vi "XDSBMPread.vi"() -> ()   [LabVIEW 2013]
panel:
  out "new picture":picture caption="new bmp"
  in  "stop":bool
  in  "base path":path=path "C:/Users/Administrator/Desktop/新建文件夹 (2)"
  in  "file name":string="a"
  # "1.This vi can read the picture of the osc screen by LAN"
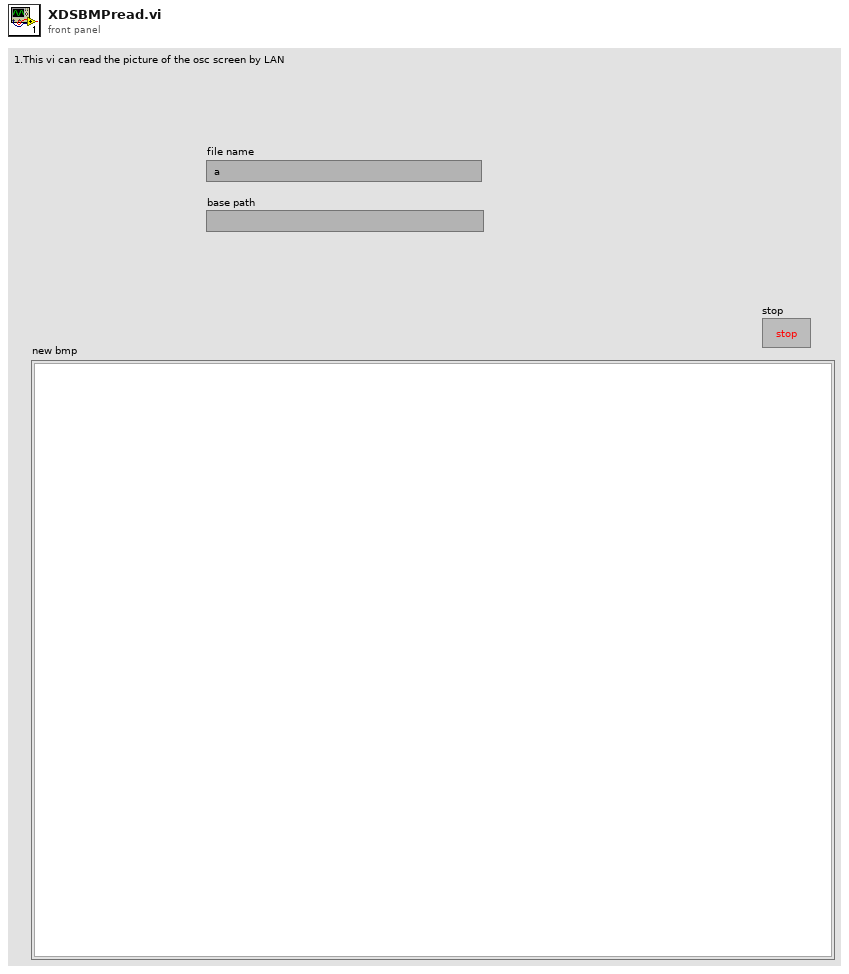
[diagram p1: front panel]
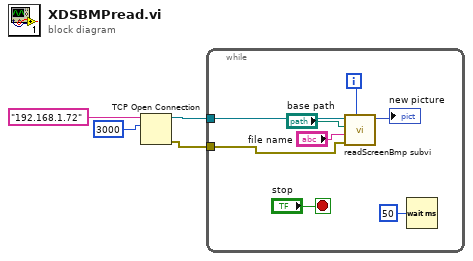
[diagram p0: block diagram]
diagram:
  n1 = TCP Open Connection(address="192.168.1.72", remote port or service name=u16 3000) -> (connection ID=w2:refnum<k5>, error out=w1:errorcluster)  [unwired: 3 in]
  n2 = while {
    tunnel: w2 -> [w8]
    tunnel: w1 -> [w7]
    i -> [w12]
    stop <- "stop" stop-if-true
    n3 = call "readScreenBmp subvi.vi"("Numeric"=w12, "error in (no error)"=w7, "file name"="file name", "base path"="base path", "TCP Network Connection in"=w8) -> ("new picture"=→"new picture":picture)  [unwired: 6 in]
    n4 = Wait (ms)(milliseconds to wait=u32 50 ("等待时间（毫秒）")) -> ()  [unwired: 1 out]
  }
